vi "DFD 2-Band Filter Bank Reconstruction with State (Array).vi"(6 "state in":cluster{"state ":dbl[]}[](array[cluster]), 7 "init? (F)":bool, 8 "error in (no error)":errorcluster, 9 "synthesis bank":T1={"mBank_Filters"=[], " mBank_#Bands"=2, "mBank_ProcMethod"=enum."General", "mBank_Coeffs"=[], "mBank_Gain"=1.0, "mBank_Type"=0} {"mBank_Type" items=["Uniform", "Non-Uniform"]; "mBank_Filters"."mMRate_SumWl" min=1 max=32 step=1; "mBank_Filters"."mMRate_InputIwl" min=1 max=32 step=1; "mBank_Filters"."mMRate_GainWl" min=1 max=32 step=1; "mBank_Filters"."mMRate_OutputWl" min=1 max=32 step=1; "mBank_Filters"."mMRate_InputWl" min=1 max=32 step=1; "mBank_Filters"."mMRate_CoefWl" min=1 max=32 step=1; "mBank_Filters"."mMRate_Mode" items=["Default"=-1, "No Rate Change"=0, "Interpolation"=1, "Decimation"=2, "Interpolated"=3, "Rational"=4]}, 10 "highpass band":dbl[](array[numeric]), 11 "lowpass band":dbl[](array[numeric])) -> (0 "error out":errorcluster, 3 "y":dbl[](array[numeric]), 4 "state out":cluster{"state ":dbl[]}[](array[cluster]))   [LabVIEW 2017, in "NI_DigFilter_FilterBank.lvlib"]
doc: "Reconstructs signal from <B>lowpass channel</B> and <B>highpass channel</B> using a 2-band synthesis bank specified by <B>synthesis bank</B>. You must specify the most recent internal input states <B>state in</B> to get the correct output. \n\n<B>state out</B> contains the most recent internal output states, which can be used as <B>state in</B> for next call to this VI if you want to process the data continuously.\n\nYou can call the VIs in <B>Filter Bank Design</B> sub-palette to design a filter bank."
uses:
  <vilib>/addons/Digital Filter Design/NI_DigFilter_FilterBank.lvlib
  <vilib>/addons/Digital Filter Design/FilterBank.llb/Object/DFD Bank Obj.ctl
  <vilib>/addons/Digital Filter Design/_Objects.llb/DFD Multirate Filter Obj.ctl
  <vilib>/addons/Digital Filter Design/_Objects.llb/DFD Multirate Mode.ctl
  <vilib>/addons/Digital Filter Design/_Objects.llb/DFD Coef Norm Type.ctl
  <vilib>/addons/Digital Filter Design/_Objects.llb/DFD Round-off Mode.ctl
  <vilib>/addons/Digital Filter Design/_Objects.llb/DFD FXP MRate Multiply Mode.ctl
  <vilib>/addons/Digital Filter Design/FilterBank.llb/Object/DFD Filter Bank Processing Method.ctl
  <vilib>/addons/Digital Filter Design/FilterBank.llb/Object/DFD Filter Bank Type.ctl
  <vilib>/addons/Digital Filter Design/NI_DigFilterLicensed.lvlib
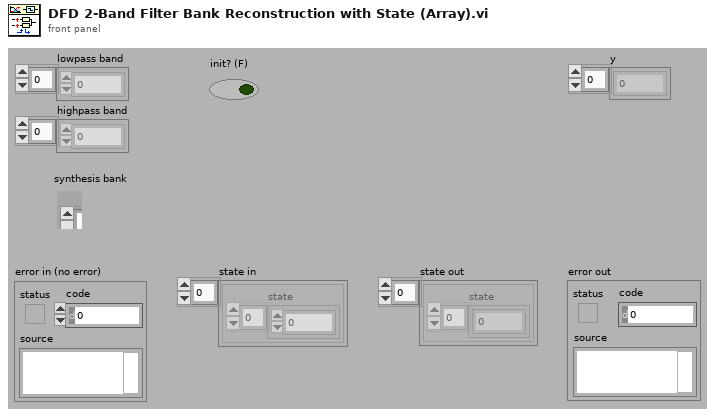
[diagram p1: front panel]
types:
  T1 = typedef "NI_DigFilter_FilterBank.lvlib/DFD Bank Obj.ctl" = cluster{"mBank_Filters":T2[], " mBank_#Bands":i32, "mBank_ProcMethod":T7, "mBank_Coeffs":dbl[], "mBank_Gain":dbl, "mBank_Type":T8}
  T2 = typedef "NI_DigFilterLicensed.lvlib/DFD Multirate Filter Obj.ctl" = cluster{"mMRate_Structure":enum16{"CIC", "FIR", "IIR", "Lattice"}, "mMRate_Mode":T3, "mMRate_Factor":i32, "mMRate_FIRParams":cluster{"mMRate_FIR_H":dbl[], "mMRate_FIR_IsNyquist?":bool, "mMRate_FIR_IsSymmetric?":bool}, "mMRate_CICParams":cluster{"mMRate_CIC_#Stage":i32, "mMRate_CIC_Lag":i32, "mMRate_CIC_Type":enum16{"Lowpass", "Highpass"}}, "mMRate_Order":i32, "mMRate_Version":string, "mMRate_Comments":string, "mMRate_RationalFactor":cluster{"mMRate_L":i32, "mMRate_M":i32}, "mMRate_Fs":dbl, "mMRate_Quantized?":bool, "mMRate_QFilterGain":dbl, "mMRate_CoefWl":i16, "mMRate_Scaling":cluster{"mMRate_ScaleByPowerOf2?":bool, "mMRate_ScaleType":T4}, "mMRate_InputWl":i16, "mMRate_OutputWl":i16, "mMRate_OutputMode":T5, "mMRate_MultMode":T6, "mMRate_BitPruning":bool, "mMRate_GainWl":i16, "mMRate_OutputFwl":i16, "mMRate_SumIwl":i16, "mMRate_InputIwl ":i16, "mMRate_SumWl":i16, "mMRate_CoefIwl":i16}
  T3 = typedef "NI_DigFilterLicensed.lvlib/DFD Multirate Mode.ctl" = i16
  T4 = typedef "NI_DigFilterLicensed.lvlib/DFD Coef Norm Type.ctl" = enum16{"No Norm", "Time Domain 1-Norm", "Time Domain 2-Norm", "Time Domain Inf-Norm"}
  T5 = typedef "NI_DigFilterLicensed.lvlib/DFD Round-off Mode.ctl" = enum16{"Nearest", "Truncation"}
  T6 = typedef "NI_DigFilterLicensed.lvlib/DFD FXP MRate Multiply Mode.ctl" = enum16{"Truncated", "Full"}
  T7 = typedef "NI_DigFilter_FilterBank.lvlib/DFD Filter Bank Processing Method.ctl" = enum16{"General", "2-Band QMF Lattice", "Cosine-Modulated"}
  T8 = typedef "NI_DigFilter_FilterBank.lvlib/DFD Filter Bank Type.ctl" = u16
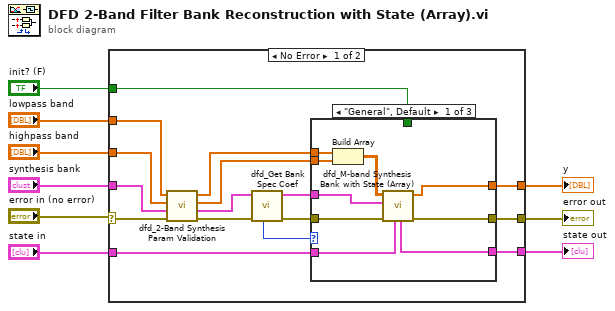
[diagram p0: block diagram]
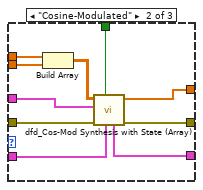
[diagram p2: hidden frame]
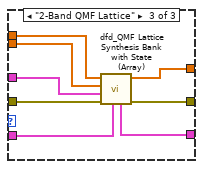
[diagram p3: hidden frame]
diagram:
  n1 = case shown="No Error" "error in (no error)" {
    selector: "error in (no error)" -> [w19 w53]
    tunnel: "synthesis bank" -> [w20 _]
    tunnel: "state in" -> [w24 _]
    tunnel: "lowpass band" -> [w22 _]
    tunnel: [w25 _] -> w4
    tunnel: [w16 w53] -> w8
    tunnel: "highpass band" -> [w21 _]
    tunnel: [w23 _] -> w2
    tunnel: "init? (F)" -> [w15 _]
    frame No Error {
      n2 = call <vilib>:"dfd_2-Band Synthesis Param Validation.vi"("error in (no error)"=w19, "filter bank"=w20, "highpass channel"=w21, "lowpass channel"=w22) -> ("error out"=w14:errorcluster, "dup filter bank"=w10:T1, "dup highpass channel"=w17:dbl[], "dup lowpass channel"=w18:dbl[])  [unwired: 4 in]
      n3 = call <vilib>:"dfd_Get Bank Spec Coef.vi"("error in (no error)"=w14, "bank in"=w10) -> ("error out"=w13:errorcluster, "bank out"=w11:T1, "processing method"=w12:T7)  [unwired: 4 in, 3 out]
      n4 = case shown="\"General\", Default" w12 {
        tunnel: w18 -> [w32 w38 w47]
        tunnel: w13 -> [w34 w44 w52]
        tunnel: [w33 w43 w49] -> w16
        tunnel: [w30 w40 w50] -> w25
        tunnel: w24 -> [w31 w41 w51]
        tunnel: [w29 w39 w48] -> w23
        tunnel: w11 -> [w26 w42 w45]
        tunnel: w17 -> [w28 w37 w46]
        tunnel: w15 -> [_ w35 _]
        frame "General", Default {
          n5 = Build Array(w32, w28) -> (w27:dbl[][])
          n6 = call <vilib>:"dfd_M-band Synthesis Bank with State (Array).vi"("state in"=w31, "error in (no error)"=w34, "filter bank in"=w26, "x"=w27) -> ("error out"=w33:errorcluster, "y"=w29:dbl[], "state out"=w30:cluster{"state ":dbl[]}[])  [unwired: 5 in]
        }
        frame "Cosine-Modulated" {
          n7 = Build Array(w38, w37) -> (w36:dbl[][])
          n8 = call <vilib>:"dfd_Cos-Mod Synthesis with State (Array).vi"("state in"=w41, "init?"=w35, "error in (no error)"=w44, "synthesis bank"=w42, "x"=w36) -> ("error out"=w43:errorcluster, "y"=w39:dbl[], "state out"=w40:cluster{"state ":dbl[]}[])  [unwired: 4 in]
        }
        frame "2-Band QMF Lattice" {
          n9 = call <vilib>:"dfd_QMF Lattice Synthesis Bank with State (Array).vi"("state in"=w51, "error in (no error)"=w52, "filter bank"=w45, "x 2"=w46, "x1"=w47) -> ("error out"=w49:errorcluster, "y1"=w48:dbl[], "state out"=w50:cluster{dbl[]}[])  [unwired: 4 in]
        }
      }
    }
    frame Error {
    }
  }
  "y" <- w2
  "error out" <- w8
  "state out" <- w4
